vi "check_placable.vi"(11 "input plate":u8[][](array[numeric])) -> (3 "placable plate":u32[][](array[numeric]))   [LabVIEW 2024]
panel:
  out "End?":bool
  in  "buf block style":u8[](array[numeric])
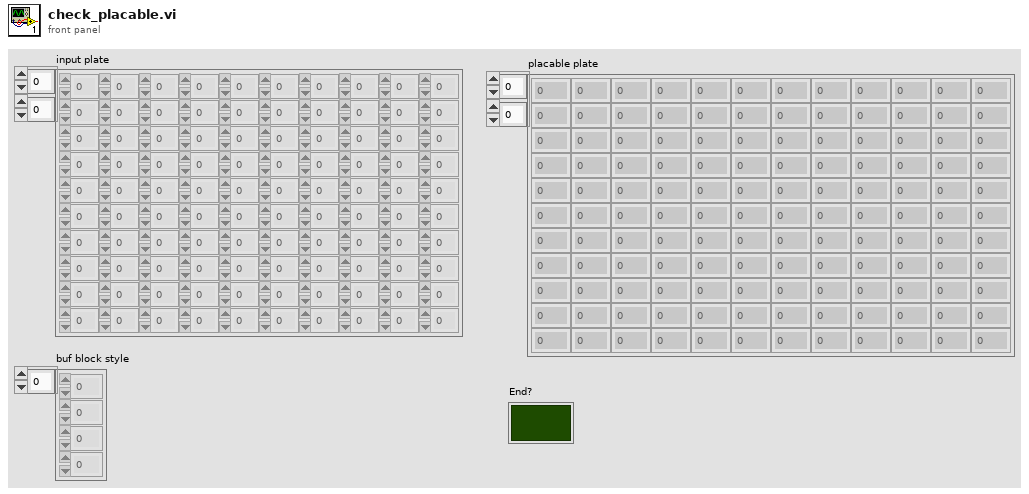
[diagram p1: front panel]
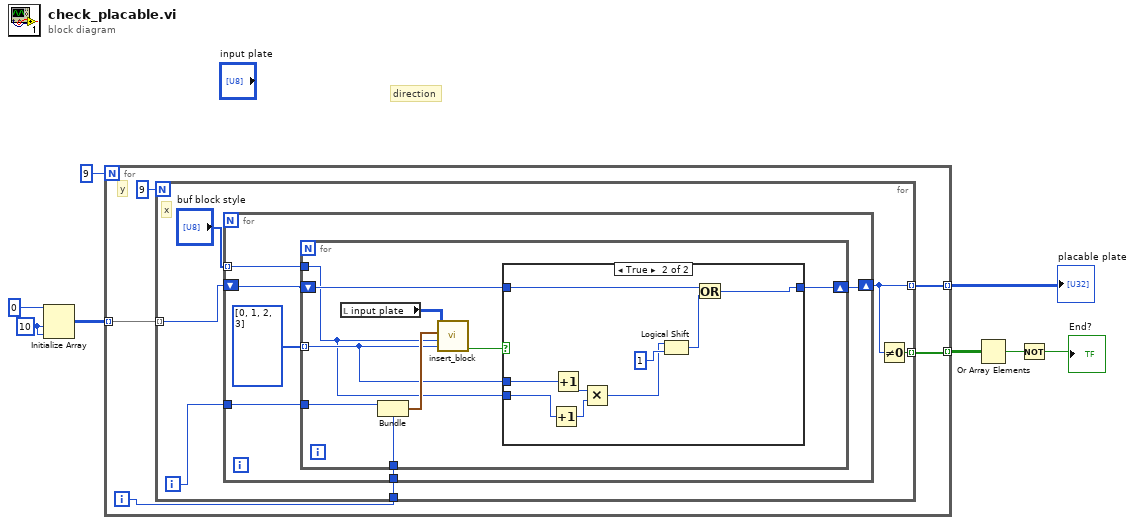
[diagram p0: block diagram]
diagram:
  w8 = 10 ("dimension size")
  # "direction"
  n1 = Initialize Array(u32 0 ("element"), w8, w8) -> (w5:u32[][])
  n2 = for {
    N: 9 -> [_]
    tunnel: w5 -> [w12] mode=indexing
    tunnel: [w10] -> w4 mode=indexing
    tunnel: [w9] -> w3 mode=indexing
    i -> [w11]
    # "y"
    n3 = for {
      N: 9 -> [_]
      tunnel: w12 -> [w19] mode=indexing
      tunnel: w11 -> [w17]
      tunnel: [w14] -> w10 mode=indexing
      tunnel: [w15] -> w9 mode=indexing
      i -> [w18]
      # "x"
      n4 = for {
        shift-right: [w20] -> w14
        shift-left: w19 -> [w21]
        tunnel: w18 -> [w25]
        tunnel: w17 -> [w24]
        tunnel: "buf block style" -> [w22] mode=indexing
        n5 = for {
          tunnel: w25 -> [w33]
          tunnel: w24 -> [w32]
          tunnel: i32[] [0, 1, 2, 3] -> [w27] mode=indexing
          tunnel: w22 -> [w26]
          shift-right: [w30] -> w20
          shift-left: w21 -> [w29]
          n6 = local read "input plate"() -> (w34:u8[][])
          n7 = Bundle(w33, w32) -> (w31:cluster{i32, i32})  [unwired: 1 in]
          n8 = call "insert_block.vi"("direction"=w27, "block_type"=w26, "position"=w31, "plate arr"=w34) -> ("valid?"=w28:bool)  [unwired: 6 in, 1 out]
          n9 = case shown="True" w28 {
            tunnel: [w35 w44] -> w30
            tunnel: w29 -> [w35 w43]
            tunnel: w27 -> [_ w39]
            tunnel: w26 -> [_ w38]
            frame False {
            }
            frame True {
              n10 = Increment(x=w38) -> (x+1=w41:u8)
              n11 = Increment(x=w39) -> (x+1=w40:i32)
              n12 = Multiply(x=w40, y=w41) -> (x*y=w36:i32)
              n13 = Logical Shift(y=w36, x=i16 1 ("y")) -> (x << y=w42:i16)
              n14 = Or(x=w43, y=w42) -> (x .or. y?=w44:u32)
            }
          }
        }
      }
      n15 = Not Equal To 0?(x=w14) -> (x != 0?=w15:bool)
    }
  }
  "placable plate" <- w4
  n16 = Or Array Elements(Boolean array=w3) -> (logical OR=w2:bool)
  n17 = Not(x=w2) -> (.not. x?=→"End?":bool)
